vi "LVClass_CorrectionDataManager Write CorrectionDataManager.vi"(8 "error in (no error)":errorcluster, 10 "CorrectionDataManager":i32, 11 "CorrectionDataManager in":refnum<class "CorrectionDataManager.lvclass">) -> (0 "error out":errorcluster, 3 "CorrectionDataManager out":refnum<class "CorrectionDataManager.lvclass">)   [LabVIEW 2020, in "CorrectionDataManager.lvclass"]
uses:
  CorrectionDataManager.lvclass
  Handle creation.ctl
  CorrectionDataManager.lvclass/CorrectionDataManager.ctl
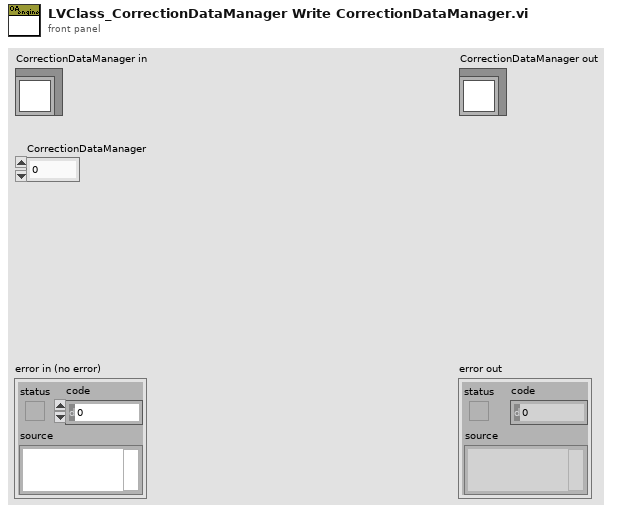
[diagram p1: front panel]
types:
  T1 = typedef "Handle creation.ctl" = enum16{"By ctor", "By write function"}
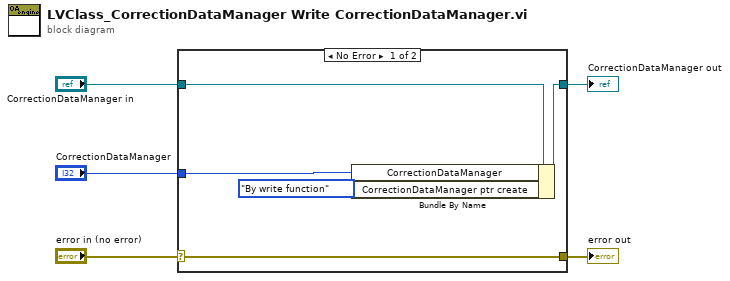
[diagram p0: block diagram]
diagram:
  n1 = case shown="No Error" "error in (no error)" {
    selector: "error in (no error)" -> [w10 w11]
    tunnel: [w10 w11] -> w4
    tunnel: [w8 w12] -> w2
    tunnel: "CorrectionDataManager in" -> [w9 w12]
    tunnel: "CorrectionDataManager" -> [w7 _]
    frame No Error {
      n2 = Bundle By Name(cluster=w9, "CorrectionDataManager"=w7, "CorrectionDataManager ptr create"=Handle_creation."By write function") -> (w8:refnum<class "CorrectionDataManager.lvclass">)
    }
    frame Error {
    }
  }
  "error out" <- w4
  "CorrectionDataManager out" <- w2
